vi "Global vab.vi"() -> ()   [LabVIEW 2015]
panel:
  out "Position (mm)":dbl
  out "Ccurrent times":dbl
  in  "Lock":bool
  out "Signal (A)":dbl format="%#_6p"
  out "Step time (ms)":u32
  # "Lock information"
  # "SM motor information"
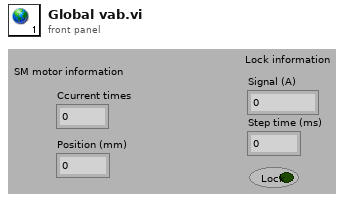
[diagram p1: front panel]
diagram:
